vi "C867_Create_JSON.vi"(8 "error in":errorcluster caption="entrée d'erreur") -> (0 "error out":errorcluster caption="sortie d'erreur", 1 "return code":i32 caption="code de retour")   [LabVIEW 2026]
uses:
  Controls/TypeDef_FGV.ctl
panel:
  out "chaîne concaténée 2":string
  out "standard error":string caption="erreur standard"
  out "standard output":string caption="sortie standard"
  out "chaîne concaténée":string
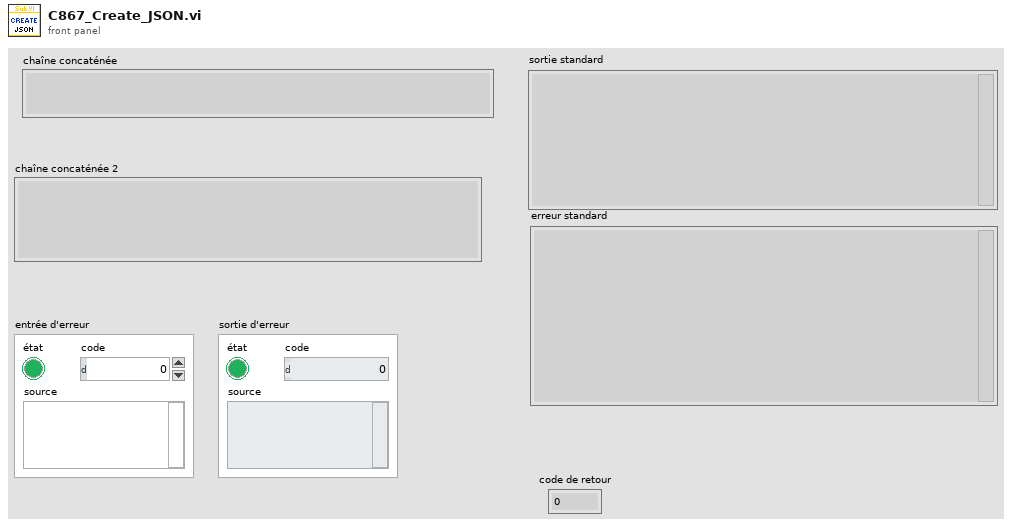
[diagram p1: front panel]
types:
  T1 = typedef "TypeDef_FGV.ctl" = enum16{"Initialize", "Write", "Read"}
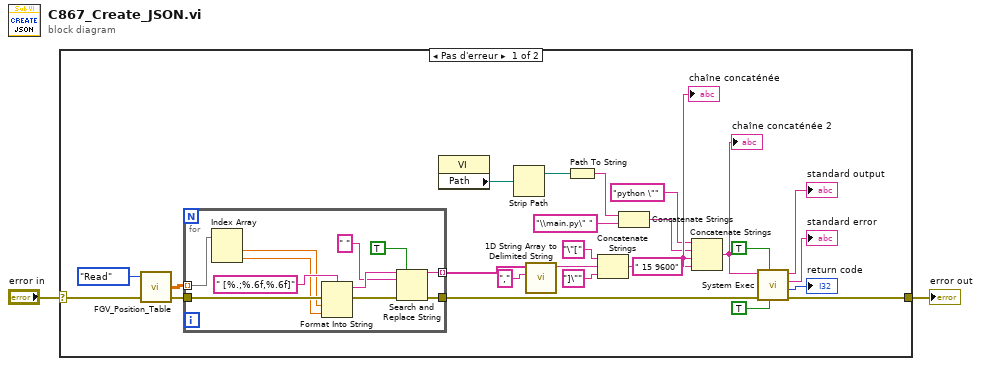
[diagram p0: block diagram]
diagram:
  n1 = case shown="Pas d'erreur" "error in" {
    selector: "error in" -> [w27 w39]
    tunnel: [w11 w39] -> w1
    frame No Error {
      n2 = call "FGV_Position_Table.vi"("error in"=w27, "Action"=TypeDef_FGV."Read") -> ("error out"=w26:errorcluster, "Position table"=w25:dbl[][])  [unwired: 1 in, 1 out]
      n3 = for {
        tunnel: w25 -> [w38] mode=indexing
        tunnel: w26 -> [w36]
        tunnel: [w32] -> w23 mode=indexing
        tunnel: [w30] -> w18
        n4 = Index Array(array=w38) -> (element #1=w35:dbl, element #2=w34:dbl)  [unwired: 2 in]
        n5 = Format Into String(format string=" [%.;%.6f,%.6f]" ("chaîne de format"), error in=w36, w35, w34) -> (resulting string=w33:string, error out=w31:errorcluster)  [unwired: 1 in]
        n6 = Search and Replace String(replace all?=TRUE ("tout remplacer ? (F)"), input string=w33, search string=" " ("chaîne recherchée"), error in=w31) -> (result string=w32:string, error out=w30:errorcluster)  [unwired: 4 in, 2 out]
      }
      n7 = property class="VI"() -> ("Path"=w8:path)  [unwired: 2 in, 2 out]
      n8 = Strip Path(path=w8) -> (stripped path=w9:path)  [unwired: 1 out]
      n9 = call <vilib>:"1D String Array to Delimited String.vi"("delimiter"=",", "string array"=w23) -> ("delimited string"=w21:string)  [unwired: 9 in]
      n10 = Path To String(path=w9) -> (string=w7:string)
      n11 = Concatenate Strings("\"[" ("chaîne"), w21, "]\"" ("chaîne")) -> (w17:string)
      "chaîne concaténée" <- w17
      n12 = Concatenate Strings(w7, "\\main.py\" " ("string")) -> (w4:string)
      n13 = Concatenate Strings("python \"" ("string"), w4, w17, " 15 9600" ("chaîne")) -> (w16:string)
      "chaîne concaténée 2" <- w16
      n14 = call <vilib>:"System Exec.vi"("run minimized? (F)"=TRUE, "wait until completion? (T)"=TRUE, "error in (no error)"=w18, "command line"=w16) -> ("error out"=w11:errorcluster, "return code"=→"return code":i32, "standard error"=→"standard error":string, "standard output"=→"standard output":string)  [unwired: 4 in]
    }
    frame Error {
    }
  }
  "error out" <- w1
